vi "SPIM_Video.vi"() -> ()   [LabVIEW 2012]
panel:
  in  "x":dbl=3.0
  out "Filter Names":string[](array[string])=["DV Video Encoder", "MJPEG Compressor"]
  in  "Convert":bool
  out "Progress":u8(slide)=99 scale=0.0..100.0
  in  "Destination Path 2":path=path "H:/P13_.AVI"
  out "Total Frames":i32=200
  out "Image":T1(plugin-control)
  out "error out":errorcluster
  in  "Source Path":path=path "D:/BackUp Data/zb-20x-new_S16_head_700mV_GCamp.ps"
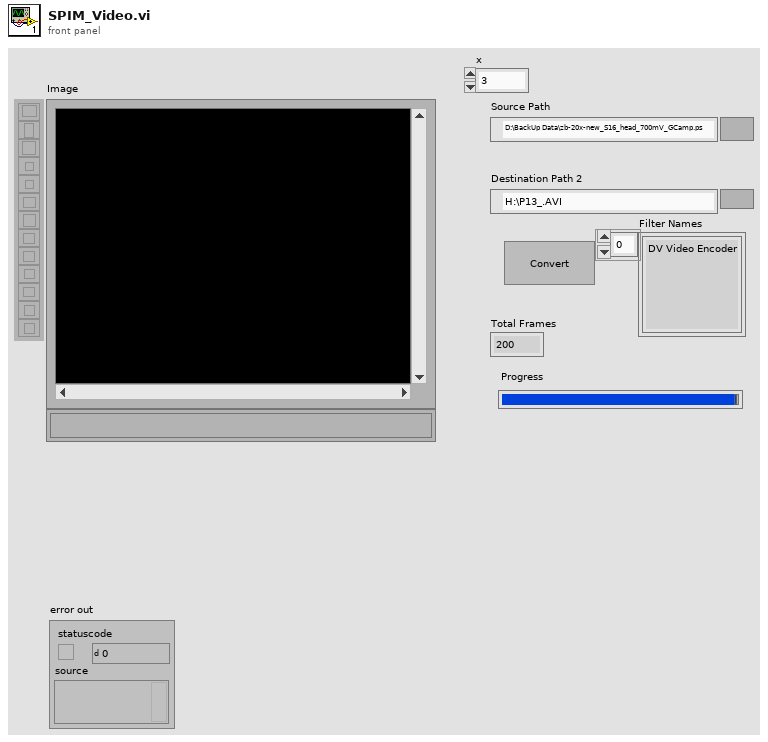
[diagram p1: front panel]
types:
  T1 = typedef "IMAQ Image.ctl" = refnum<image>
  T2 = typedef "Image Type" = u32
  T3 = typedef "AviRefnum.ctl" = refnum<k1>
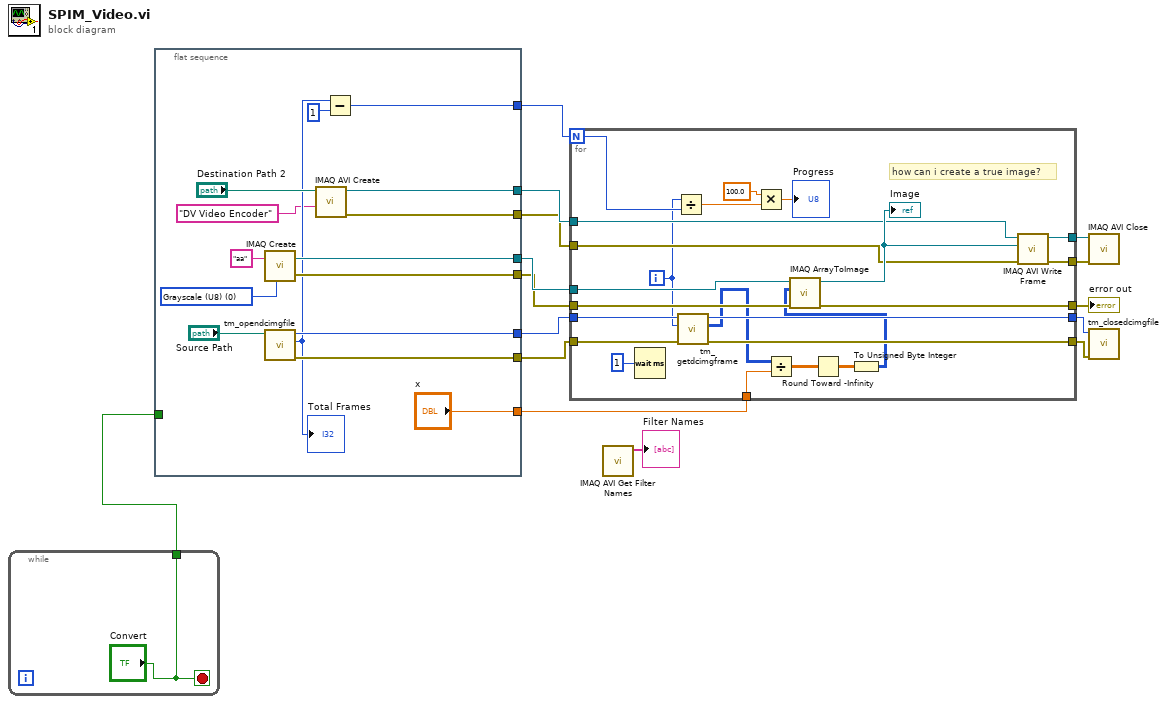
[diagram p0: block diagram]
diagram:
  n1 = while {
    tunnel: ["Convert"] -> w2
    stop <- "Convert" stop-if-true
  }
  n2 = flat-sequence {
    tunnel: [w29] -> w15
    tunnel: [w28] -> w13
    tunnel: [w26] -> w12
    tunnel: [w25] -> w11
    tunnel: [w23] -> w8
    tunnel: [w22] -> w7
    tunnel: [w19] -> w4
    tunnel: w2 -> [_]
    tunnel: ["x"] -> w1
    frame #0 {
      w27 = T2 0 items=["Grayscale (U8)", "Grayscale (I16)", "Grayscale (SGL)", "Complex (CSG)", "RGB (U32)", "HSL (U32)", "RGB (U64)"] ("Image Type")
      n3 = call "IMAQ Create"("Image Name"="aa", "Image Type"=w27) -> ("New Image"=w29:T1, "error out"=w28:errorcluster)  [unwired: 3 in]
      n4 = call <userlib>:"tm_opendcimgfile.vi"("Path"="Source Path") -> ("error out"=w25:errorcluster, "Total Frames"=w21:i32, "File Handle"=w26:u32)  [unwired: 8 in]
      "Total Frames" <- w21
      n5 = call "IMAQ AVI Create"("Compression Filter"="DV Video Encoder", "AVI Path"="Destination Path 2") -> ("error out"=w22:errorcluster, "Avi Refnum"=w23:T3)  [unwired: 8 in]
      n6 = Subtract(x=w21, y=1) -> (x-y=w19:i32)
    }
  }
  n7 = for {
    N: w4 -> [w41]
    tunnel: w15 -> [w54]
    tunnel: [w53] -> w14
    tunnel: w13 -> [w52]
    tunnel: w12 -> [w51]
    tunnel: w11 -> [w50]
    tunnel: [w48] -> w10
    tunnel: [w47] -> w9
    tunnel: w8 -> [w45]
    tunnel: w7 -> [w44]
    tunnel: [w43] -> w6
    tunnel: [w42] -> w5
    tunnel: w1 -> [w32]
    i -> [w40]
    # "how can i create a true image?"
    n8 = Wait (ms)(milliseconds to wait=u32 1) -> ()  [unwired: 1 out]
    n9 = Divide(x=w40, y=w41) -> (x/y=w38:dbl)
    n10 = call <userlib>:"tm_getdcimgframe.vi"("error in (no error)"=w50, "Frame Index"=w40, "File Handle in"=w51) -> ("error out"=w47:errorcluster, "Data"=w36:u16[][], "File Handle out"=w48:u32)  [unwired: 5 in, 1 out]
    n11 = Multiply(x=100.0, y=w38) -> (x*y=→"Progress":dbl)
    n12 = Divide(x=w36, y=w32) -> (x/y=w35:dbl[][])
    n13 = Round Toward -Infinity(1:w35) -> (0:w34:dbl[][])
    n14 = To Unsigned Byte Integer(number=w34) -> (unsigned 8bit integer=w33:u8[][])
    n15 = call "IMAQ ArrayToImage"("error in (no error)"=w52, "Image Pixels (U8)"=w33, "Image"=w54) -> ("error out"=w53:errorcluster, "Image Out"=w46:T1)  [unwired: 7 in]
    "Image" <- w46
    n16 = call "IMAQ AVI Write Frame"("error in (no error)"=w44, "Image"=w46, "Avi Refnum"=w45) -> ("error out"=w42:errorcluster, "Avi Refnum (duplicate)"=w43:T3)  [unwired: 7 in]
  }
  "error out" <- w14
  n17 = call "IMAQ AVI Get Filter Names"() -> ("Filter Names"=→"Filter Names":string[])  [unwired: 10 in, 1 out]
  n18 = call "IMAQ AVI Close"("error in (no error)"=w5, "Avi Refnum"=w6) -> ()  [unwired: 9 in, 1 out]
  n19 = call <userlib>:"tm_closedcimgfile.vi"("error in (no error)"=w9, "File Handle"=w10) -> ()  [unwired: 9 in, 1 out]
